vi "Update Button State.vi"(8 "error in (no error)":errorcluster, 10 "Current Buttons":bool[](array[boolean]), 11 "Joystick in":refnum<class "Joystick.lvclass">) -> (0 "error out":errorcluster, 3 "Joystick out":refnum<class "Joystick.lvclass">)   [LabVIEW 2014, in "Joystick.lvlib" / "Joystick.lvclass"]
uses:
  Joystick.lvclass
  Joystick.lvclass/Joystick.ctl
  Button State.ctl
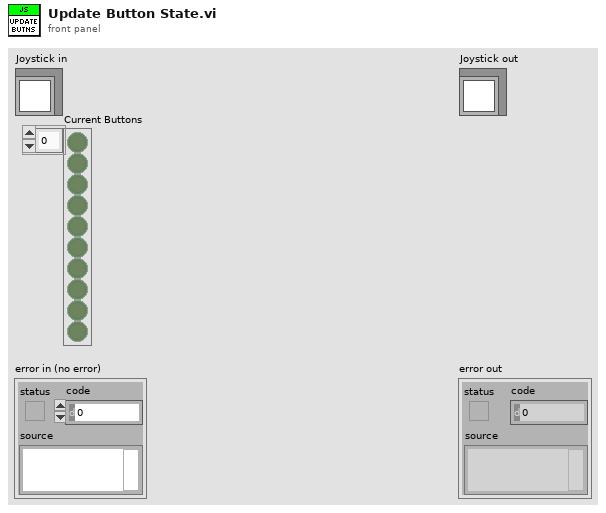
[diagram p1: front panel]
types:
  T1 = typedef "Joystick.lvlib/Joystick.lvclass/Button State.ctl" = cluster{"Pressed":bool, "Instance Name":string, "Toggled":bool, "Just Changed":bool}
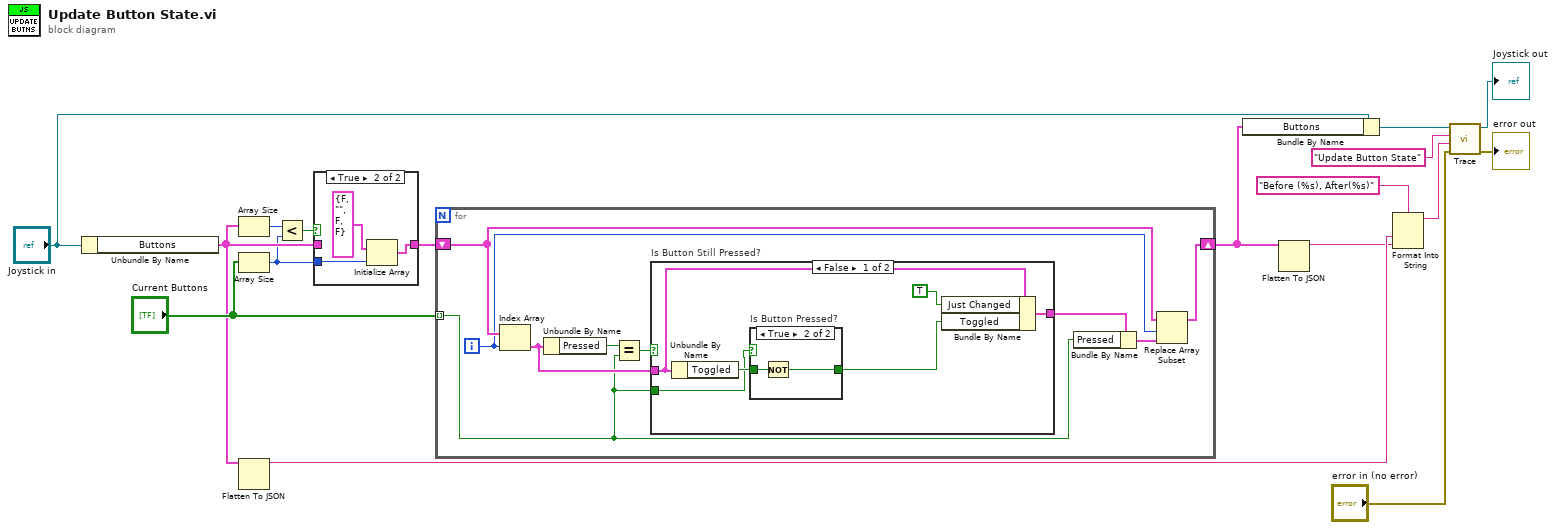
[diagram p0: block diagram]
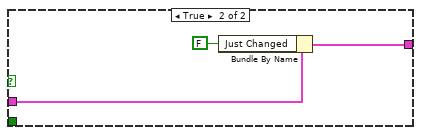
[diagram p4: hidden frame]
diagram:
  n1 = Unbundle By Name("Joystick in") -> ("Buttons"=w3:T1[])
  n2 = Array Size(array=w3) -> (size(s)=w5:i32)
  n3 = Array Size(array="Current Buttons") -> (size(s)=w2:i32)
  n4 = Flatten To JSON(anything=w3) -> (JSON string=w12:string)  [unwired: 2 in, 1 out]
  n5 = Less?(x=w5, y=w2) -> (x < y?=w4:bool)
  n6 = case shown="True" w4 {
    tunnel: w3 -> [w18 _]
    tunnel: w2 -> [_ w20]
    tunnel: [w18 w19] -> w1
    frame False {
    }
    frame True {
      n7 = Initialize Array(T1 {"Pressed"=FALSE, "Instance Name"="", "Toggled"=FALSE, "Just Changed"=FALSE} ("Button State"), w20) -> (w19:T1[])
    }
  }
  n8 = for {
    shift-right: [w27] -> w11
    shift-left: w1 -> [w28]
    tunnel: "Current Buttons" -> [w22] mode=indexing
    i -> [w24]
    n9 = Index Array(array=w28, index=w24) -> (element=w26:T1)
    n10 = Unbundle By Name(w26) -> ("Pressed"=w30:bool)
    n11 = Equal?(x=w30, y=w22) -> (x = y?=w29:bool)
    n12 = case "Is Button Still Pressed?" shown="False" w29 {
      tunnel: w26 -> [w34 w42]
      tunnel: [w36 w41] -> w25
      tunnel: w22 -> [w31 _]
      frame False {
        n13 = Unbundle By Name(w34) -> ("Toggled"=w33:bool)
        n14 = case "Is Button Pressed?" shown="True" w31 {
          tunnel: w33 -> [w37 w39]
          tunnel: [w37 w38] -> w32
          frame False {
          }
          frame True {
            n15 = Not(x=w39) -> (.not. x?=w38:bool)
          }
        }
        n16 = Bundle By Name(cluster=w34, "Just Changed"=TRUE, "Toggled"=w32) -> (w36:T1)
      }
      frame True {
        n17 = Bundle By Name(cluster=w42, "Just Changed"=FALSE) -> (w41:T1)
      }
    }
    n18 = Bundle By Name(cluster=w25, "Pressed"=w22) -> (w23:T1)
    n19 = Replace Array Subset(array=w28, new element=w23, index=w24) -> (w27:T1[])
  }
  n20 = Bundle By Name(cluster="Joystick in", "Buttons"=w11) -> (w16:refnum<class "Joystick.lvclass">)
  n21 = Flatten To JSON(anything=w11) -> (JSON string=w10:string)  [unwired: 2 in, 1 out]
  n22 = Format Into String(format string="Before (%s), After(%s)", w12, w10) -> (resulting string=w9:string)  [unwired: 2 in, 1 out]
  n23 = call-dynamic "Trace.vi"("error in (no error)"="error in (no error)", "System Message"=w9, "System Action"="Update Button State", "System Actor in"=w16) -> ("error out"=→"error out":errorcluster, "System Actor out"=→"Joystick out":refnum<class "Joystick.lvclass">)  [unwired: 6 in]
